vi "Get VI Refnum Address.vi"(1 "VI Refnum":refnum<vi>) -> (0 "Get Ref Address":u16)   [LabVIEW 2015]
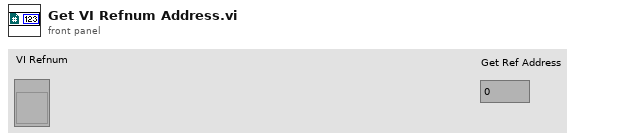
[diagram p1: front panel]
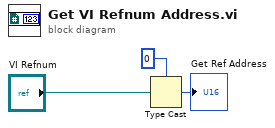
[diagram p0: block diagram]
diagram:
  n1 = Type Cast(type=u16 0, x="VI Refnum") -> (*(type *) &x=→"Get Ref Address":u16)
